vi "Filter Device List.vi"(5 "Old List":u16[](array[numeric]), 7 "New List":u16[](array[numeric]), 10 "Remove object pressed":i32, 11 "Remove object":i32) -> (2 "Filtered List":u16[](array[numeric]))   [LabVIEW 2019]
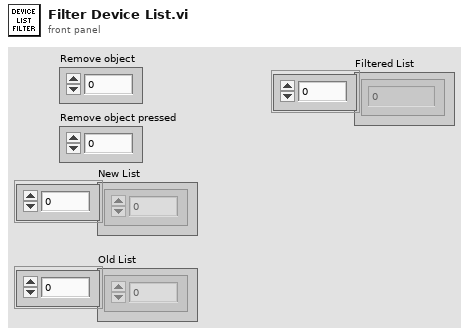
[diagram p1: front panel]
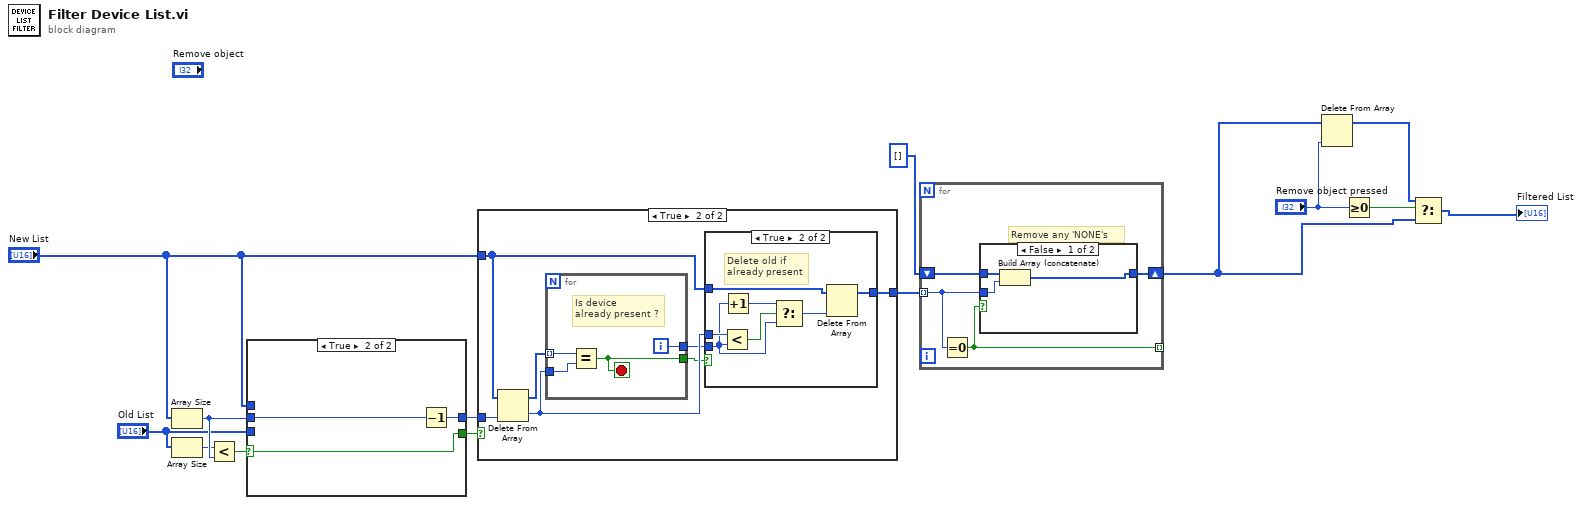
[diagram p0: block diagram]
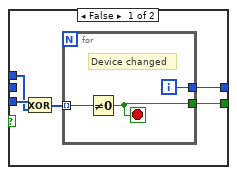
[diagram p3: hidden frame]
diagram:
  n1 = Array Size(array="New List") -> (size(s)=w12:i32)
  n2 = Array Size(array="Old List") -> (size(s)=w9:i32)
  n3 = Less?(x=w9, y=w12) -> (x < y?=w11:bool)
  n4 = case shown="True" w11 {
    selector: w11 -> [_ w23]
    tunnel: "Old List" -> [w19 _]
    tunnel: "New List" -> [w17 _]
    tunnel: [w16 w25] -> w7
    tunnel: [w15 w23] -> w8
    tunnel: w12 -> [_ w24]
    frame False {
      n5 = Exclusive Or(1:w17, 2:w19) -> (0:w18:u16[])
      n6 = for {
        tunnel: w18 -> [w20] mode=indexing
        tunnel: [w22] -> w15
        tunnel: [w21] -> w16
        i -> [w21]
        stop <- w22 stop-if-true
        # "Device changed"
        n7 = Not Equal To 0?(x=w20) -> (x != 0?=w22:bool)
      }
    }
    frame True {
      n8 = Decrement(x=w24) -> (x-1=w25:i32)
    }
  }
  n9 = case shown="True" w8 {
    tunnel: "New List" -> [w26 w31]
    tunnel: w7 -> [_ w33]
    tunnel: [w26 w27] -> w14
    frame False {
    }
    frame True {
      n10 = Delete From Array(array=w31, index=w33) -> (deleted portion=w30:u16, array with subset deleted=w32:u16[])  [unwired: 1 in]
      n11 = for {
        tunnel: w32 -> [w43] mode=indexing
        tunnel: w30 -> [w42]
        tunnel: [w45] -> w29
        tunnel: [w44] -> w28
        i -> [w44]
        stop <- w45 stop-if-true
        # "Is device\nalready present ?"
        n12 = Equal?(x=w43, y=w42) -> (x = y?=w45:bool)
      }
      n13 = case shown="True" w29 {
        tunnel: w31 -> [w34 w36]
        tunnel: w30 -> [_ w41]
        tunnel: w28 -> [_ w39]
        tunnel: [w34 w35] -> w27
        frame False {
        }
        frame True {
          # "Delete old if\nalready present"
          n14 = Less?(x=w41, y=w39) -> (x < y?=w40:bool)
          n15 = Increment(x=w39) -> (x+1=w38:i32)
          n16 = Select(t=w38, s=w40, f=w39) -> (s? t:f=w37:i32)
          n17 = Delete From Array(array=w36, index=w37) -> (array with subset deleted=w35:u16[])  [unwired: 1 in, 1 out]
        }
      }
    }
  }
  n18 = for {
    tunnel: w14 -> [w46] mode=indexing
    shift-right: [w48] -> w2
    shift-left: u16[] [] -> [w49]
    tunnel: [w47] -> _ mode=indexing
    # "Remove any 'NONE's"
    n19 = Equal To 0?(x=w46) -> (x = 0?=w47:bool)
    n20 = case shown="False" w47 {
      tunnel: w46 -> [w52 _]
      tunnel: [w51 w53] -> w48
      tunnel: w49 -> [w50 w53]
      frame False {
        n21 = Build Array (concatenate)(w50, w52) -> (w51:u16[])
      }
      frame True {
      }
    }
  }
  n22 = Delete From Array(array=w2, index="Remove object pressed") -> (array with subset deleted=w3:u16[])  [unwired: 1 in, 1 out]
  n23 = Greater Or Equal To 0?(x="Remove object pressed") -> (x >= 0?=w6:bool)
  n24 = Select(t=w3, s=w6, f=w2) -> (s? t:f=→"Filtered List":u16[])
